vi "setAllChannels.vi"(8 "error in (no error)":errorcluster, 10 "allChannelProperties":variant, 11 "Inst.Krohn-Hite-7008 in":refnum<class "Inst.Krohn-Hite-7008.lvclass">) -> (0 "error out":errorcluster, 3 "Inst.Krohn-Hite-7008 out":refnum<class "Inst.Krohn-Hite-7008.lvclass">)   [LabVIEW 2019, in "Inst.KH7008.lvlib" / "Inst.Krohn-Hite-7008.lvclass"]
uses:
  Inst.Krohn-Hite-7008.lvclass
  <userlib>/LevyLab/Instrument Framework/Instrument Types/Amplifier/Instrument.Amplifier.lvclass
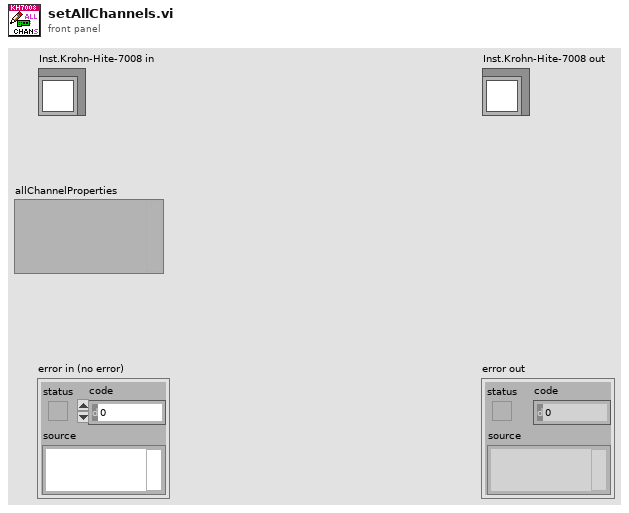
[diagram p1: front panel]
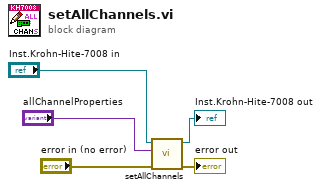
[diagram p0: block diagram]
diagram:
  n1 = call-parent "setAllChannels.vi"("error in (no error)"="error in (no error)", "allChannelProperties"="allChannelProperties", "Instrument.Amplifier in"="Inst.Krohn-Hite-7008 in") -> ("error out"=→"error out":errorcluster, "Instrument.Amplifier out"=→"Inst.Krohn-Hite-7008 out":refnum<class "Inst.Krohn-Hite-7008.lvclass">)  [unwired: 7 in]
